vi "Main.vi"() -> (0 "errout":errorcluster caption="error out")   [LabVIEW 2020]
uses:
  <vilib>/MakerHub/LINX/Private/Type Defs/LINX Ref.ctl
  <vilib>/MakerHub/LINX/Private/Type Defs/Platform.ctl
  <vilib>/MakerHub/LINX/Private/Type Defs/Interface.ctl
  <vilib>/MakerHub/LINX/Private/Device/Type Defs/LINX Device Config.ctl
  <vilib>/MakerHub/LINX/Private/Device/Type Defs/TCP Config.ctl
  <vilib>/MakerHub/LINX/Private/Device/Type Defs/Channels.ctl
  ctrl glo/nav.ctl
  <userlib>/Alex Log/Log_ligne.ctl
  ctrl glo/VG_progressBar.vi
  SubVi/Param_Sys.vi
  SubVi/Param_Stack.vi
  <instrlib>/IT6000C/IT6000C.lvlib
  <vilib>/MakerHub/LINX/LMH-LINX.lvlib
  <vilib>/MakerHub/LINX/Private/Device/Device.lvlib
panel:
  out "Config Path":string
  out "chaîne concaténée":string
  out "30?":bool=TRUE
  out "DCIR+?":bool=TRUE
  out "network out":path
  out "Ok final":bool
  out "3P4S?":bool=TRUE
  out "VISA OUT":T1
  out "UNO TAK out":T2
  out "Auto?":bool
  out "progression":u8(slide) scale=0.0..100.0
  out "fin":bool
  out "errout":errorcluster caption="sortie d'erreur"
  in  "image":string
  out "Image 2D":picture
  out "Chaîne 2":string
  out "Chaîne":string
  # "V2.3.1"
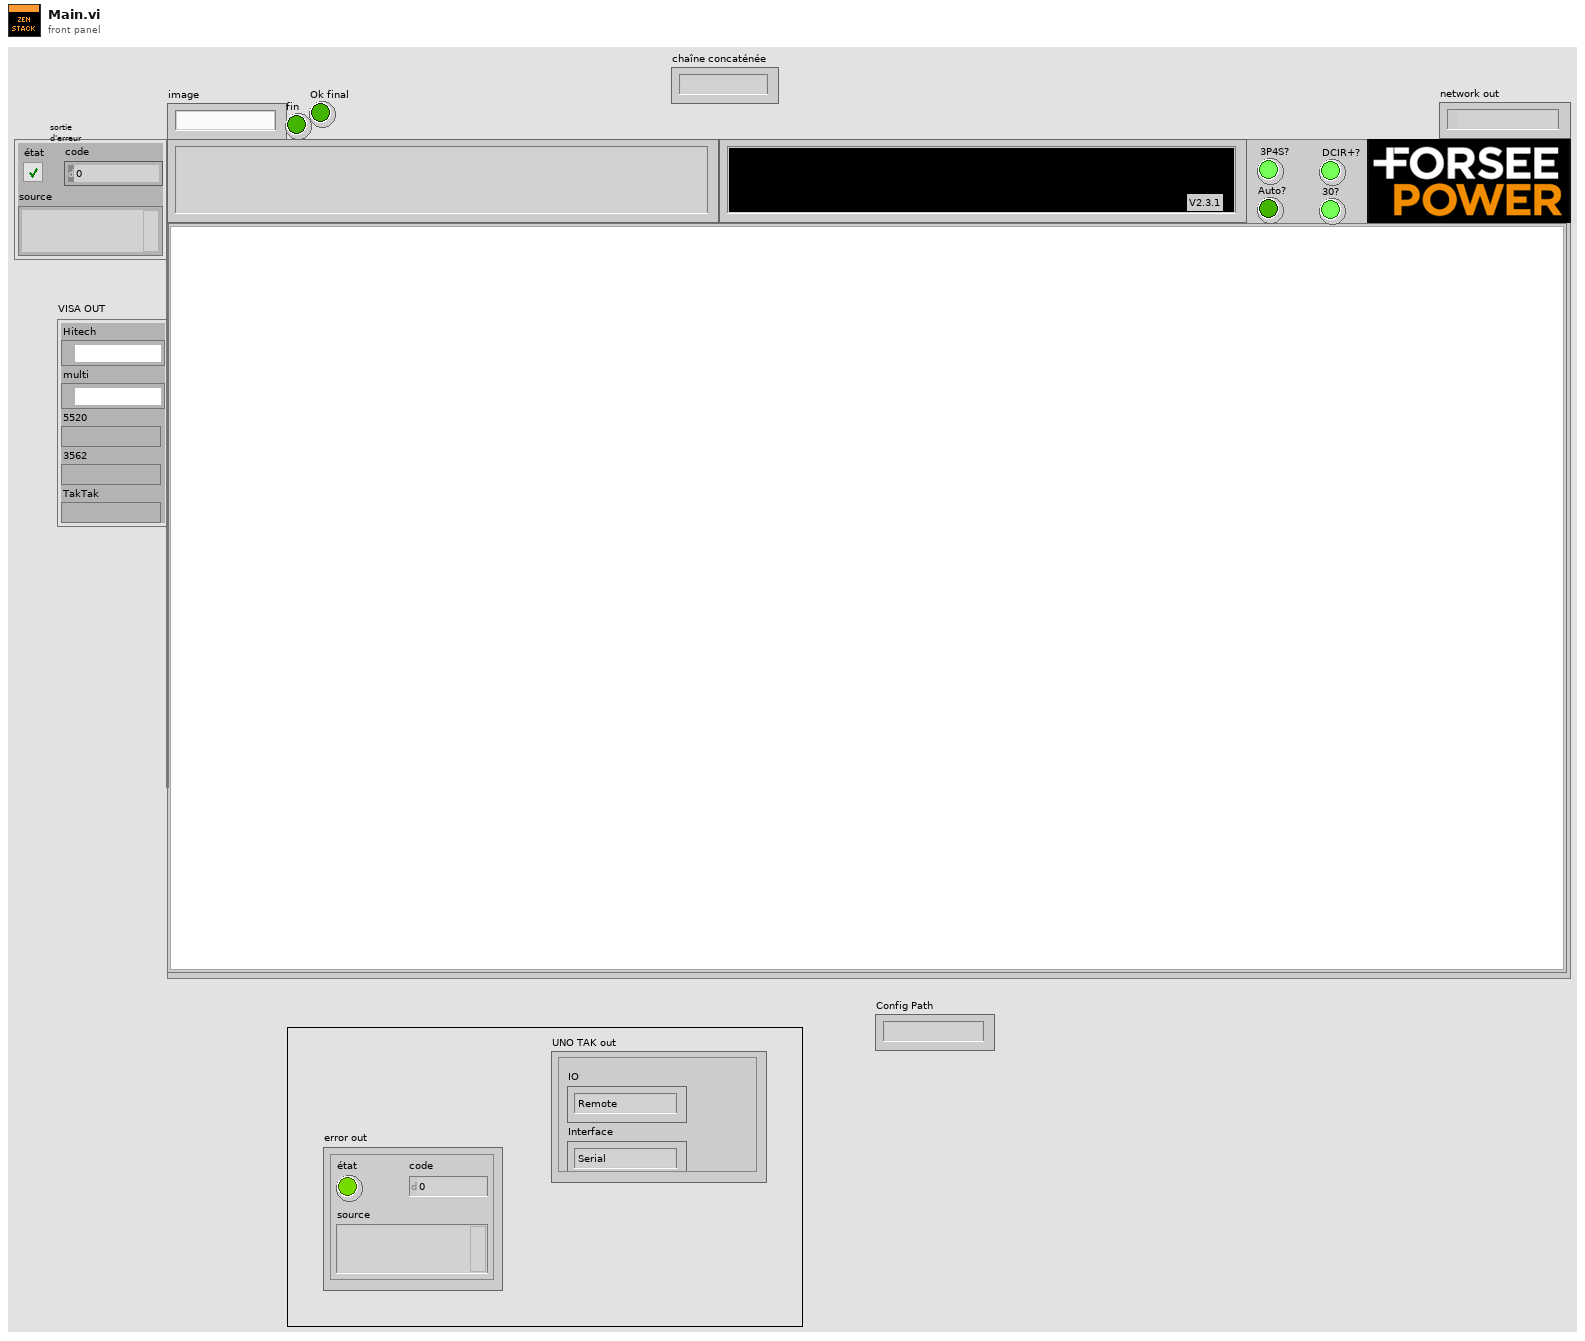
[diagram p1: front panel]
types:
  T1 = cluster{"Hitech":refnum<visa-resource-name>, "multi":refnum<visa-resource-name>, "5520":refnum<visa-resource-name>, "3562":refnum<visa-resource-name>, "TakTak":refnum<visa-resource-name>}
  T2 = typedef "LMH-LINX.lvlib/LINX Ref.ctl" = cluster{"IO":T3, "Interface":T4, "LINX Device Config":T5}
  T3 = typedef "LMH-LINX.lvlib/Platform.ctl" = enum16{"Remote", "Local"}
  T4 = typedef "LMH-LINX.lvlib/Interface.ctl" = enum16{"Serial", "TCP"}
  T5 = typedef "LMH-LINX.lvlib/Device.lvlib/LINX Device Config.ctl" = cluster{"Interface":T4, "COM Port":refnum<visa-resource-name>, "TCP Configuration":T6, "Device Family":u8, "Device ID":u8, "Device Name":string, "TCP Ref":refnum<k5>, "Channels":T7}
  T6 = typedef "LMH-LINX.lvlib/Device.lvlib/TCP Config.ctl" = cluster{"IP Address":string, "Port":u16}
  T7 = typedef "LMH-LINX.lvlib/Channels.ctl" = cluster{"DI":u8[], "DO":u8[], "AI":u8[], "AO":u8[], "PWM":u8[], "QE":u8[], "UART":u8[], "I2C 2":u8[], "SPI":u8[], "CAN":u8[], "Servo":u8[], "AI Ref (V)":dbl, "AI Resolution (Bits)":u8, "AO Ref (V)":dbl, "AO Resolution (Bits)":u8}
  T8 = typedef "nav.ctl" = enum8{"DEM0", "DEM1", "Init", "DEM2", "SCAN", "SECU", "PreDCIR", "OCVACIR", "Montage", "GoInsuPlus", "InsulationBplus", "GoInsuMoins", "InsulationBmoins", "GoDCIR", "DCIR", "Collage PAD", "Demontage", "CLOSE", "extinction", "CRASH"}
  T9 = typedef "Log_ligne.ctl" = enum16{"Def", "Volt V", "Volt mV", "ohm Ohm", "ohm mOhm", "ohm kOhm", "ohm MOhm", "Opérateur", "EPI", "SN"}
  T10 = cluster{"résolution":i16, "resu":dbl, "Type":T9, "Data in":string}
  T11 = cluster{"Baud Rate":u32, "Parity":u16, "Data Bits":u16, "Stop Bits":u16, "Flow Control":u16}
  T12 = cluster{"résolution":i16, "resu":dbl, "Type":T9, "Data in":string}[]
  T13 = cluster{"Cell1 V":sgl, "Cell2 V":sgl, "Cell3 V":sgl, "Cell4 V":sgl, "Cell1 °C":sgl, "Cell2 °C":sgl, "Cell5 V":sgl, "Cell6 V":sgl}
  T14 = typedef "imagedata.ctl" = cluster{"image type":i32, "image depth":i32, "image":u8[], "mask":u8[], "colors":u32[], "Rectangle":cluster{"left":i16, "top":i16, "right":i16, "bottom":i16}}
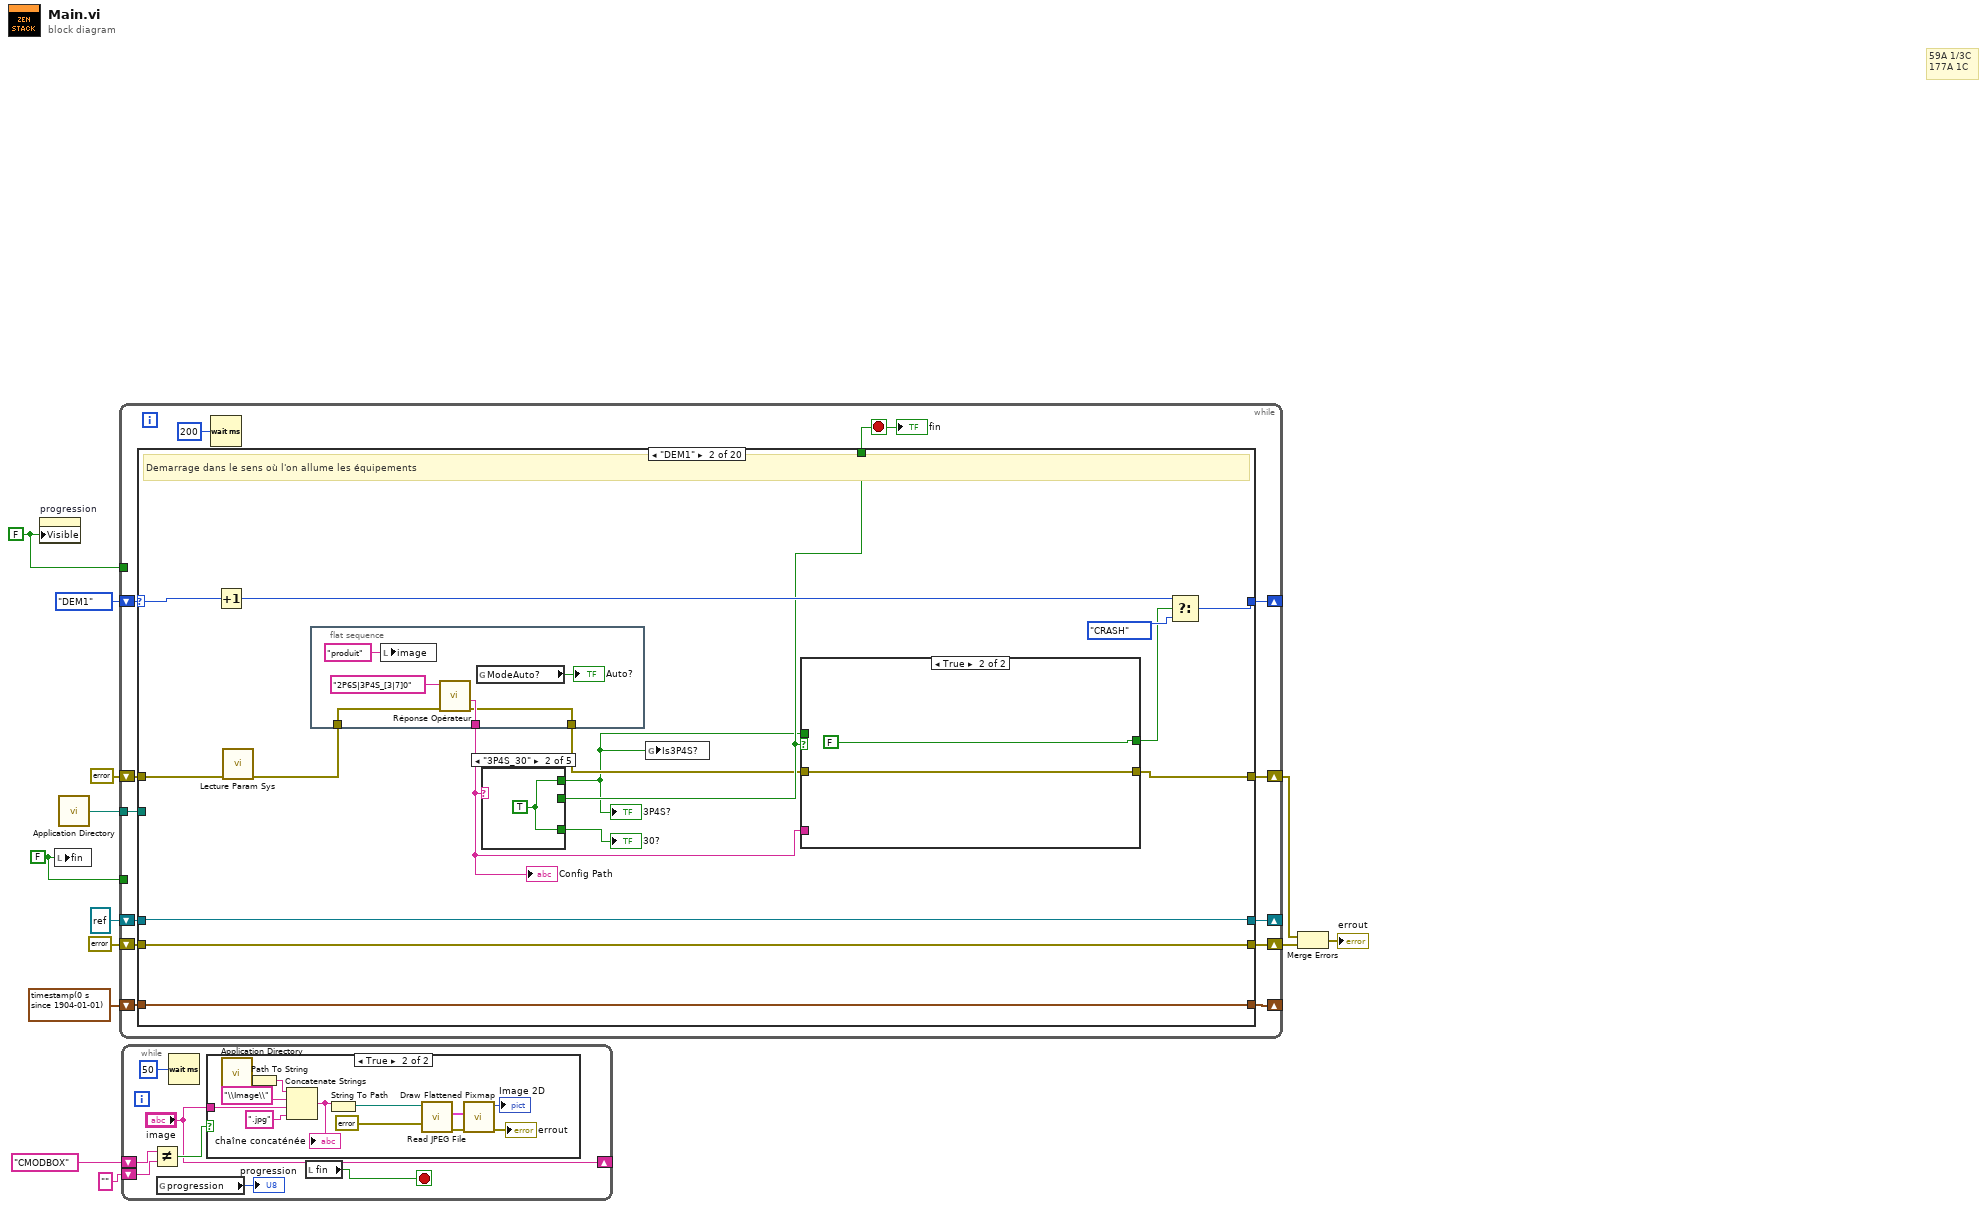
[diagram p0: block diagram]
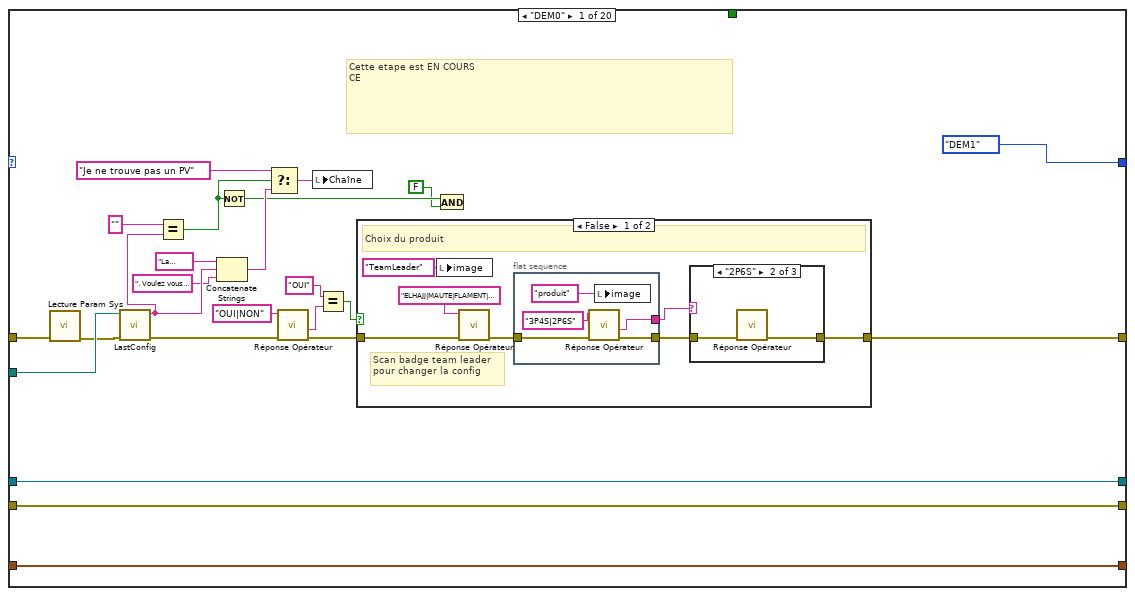
[diagram p3: hidden frame]
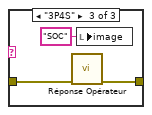
[diagram p5: hidden frame]
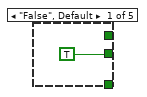
[diagram p7: hidden frame]
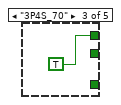
[diagram p8: hidden frame]
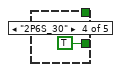
[diagram p9: hidden frame]
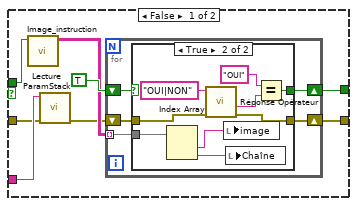
[diagram p11: hidden frame]
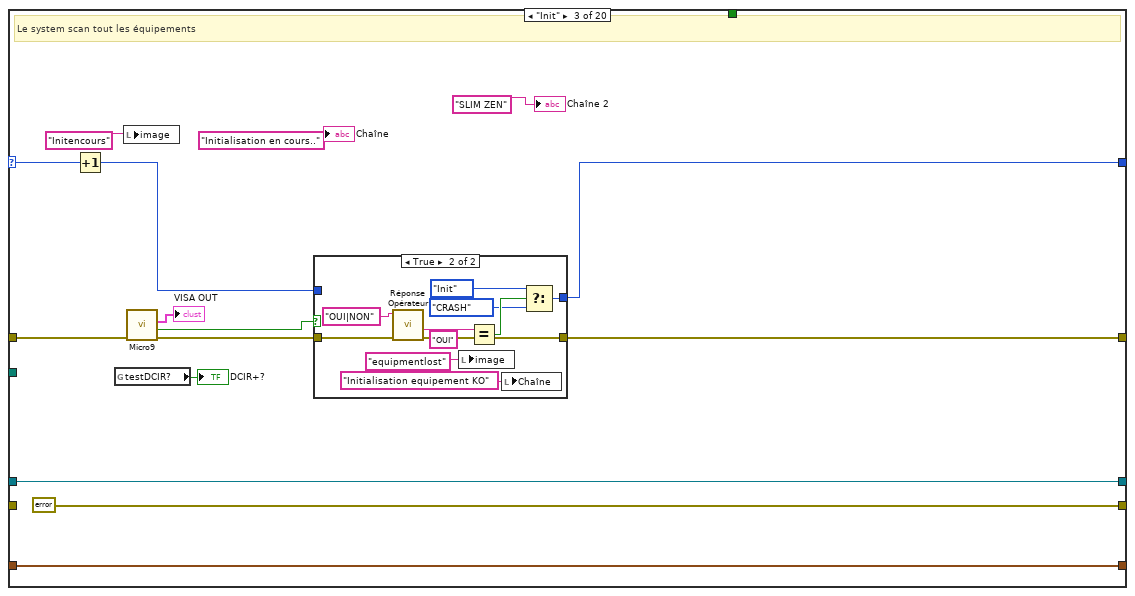
[diagram p13: hidden frame]
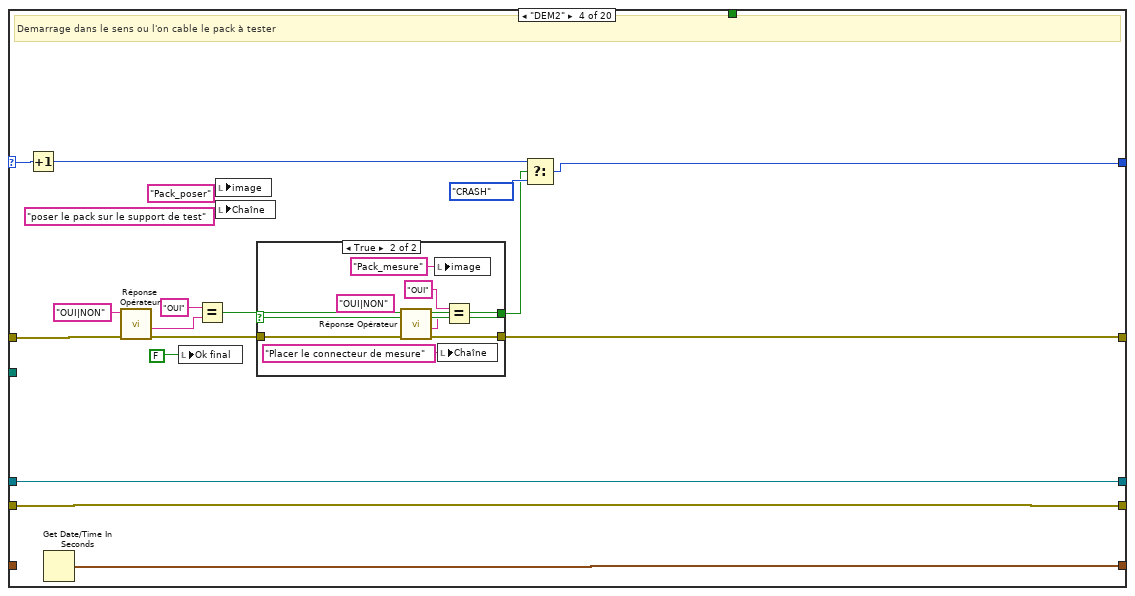
[diagram p15: hidden frame]
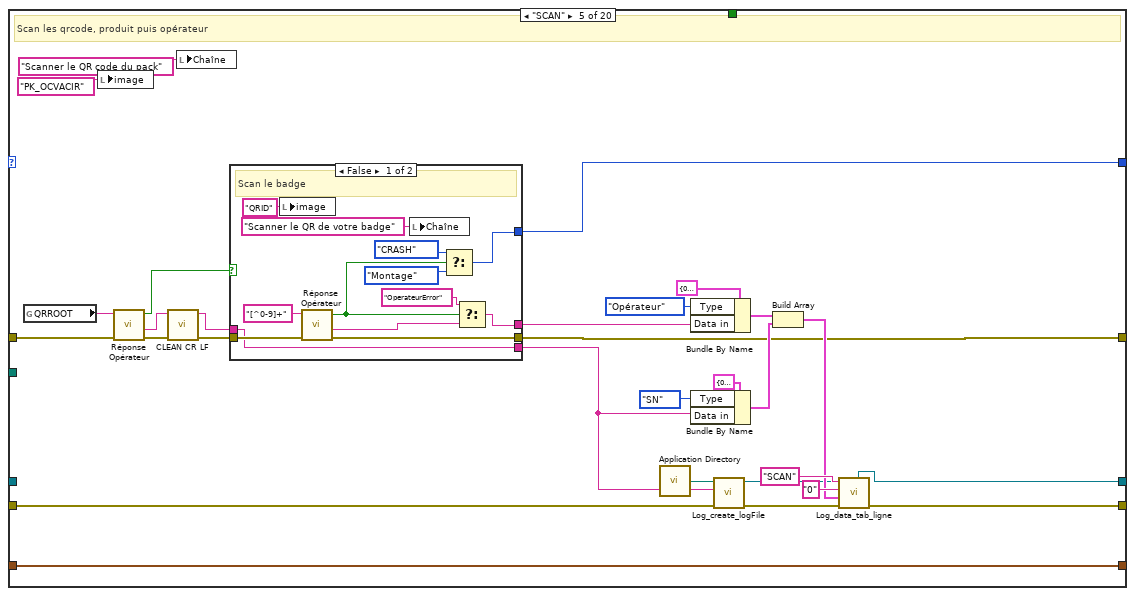
[diagram p17: hidden frame]
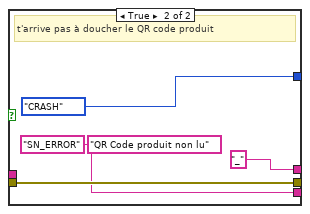
[diagram p18: hidden frame]
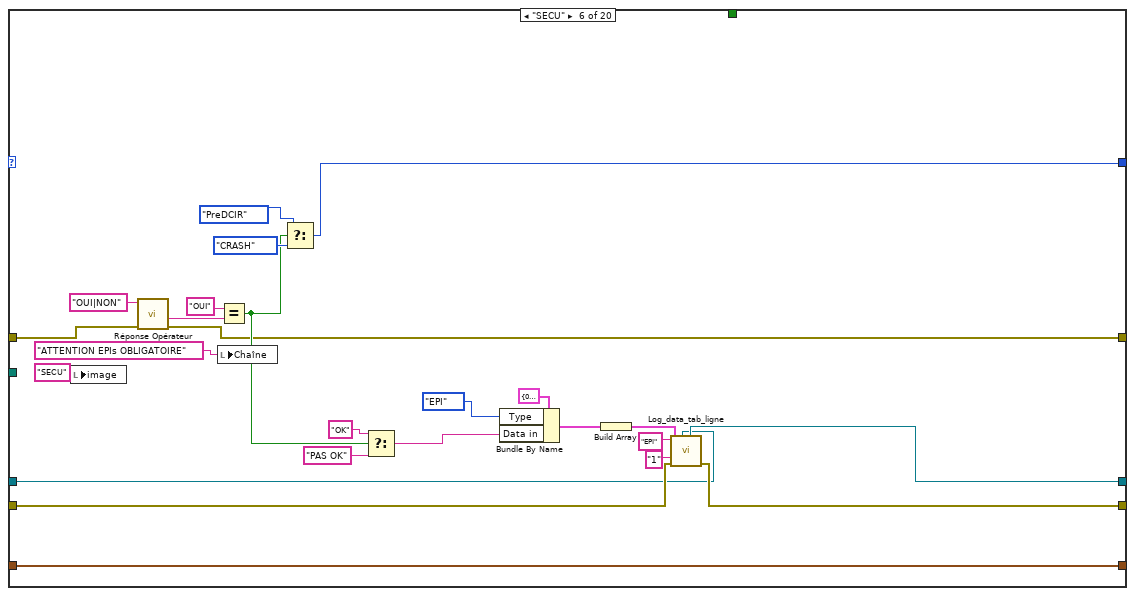
[diagram p19: hidden frame]
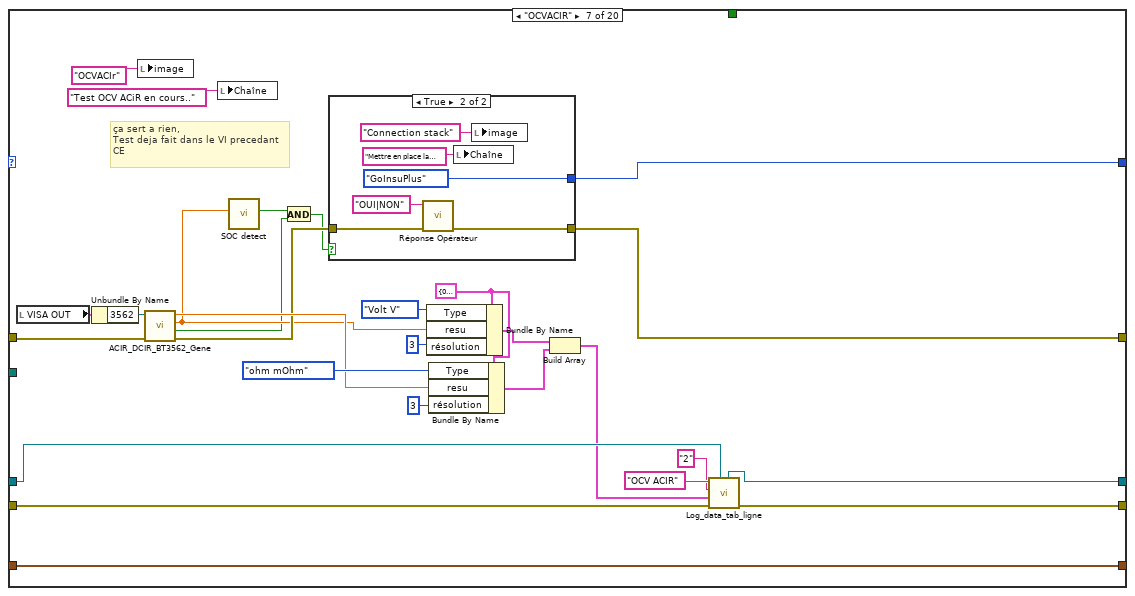
[diagram p20: hidden frame]
diagram:
  w4 = FALSE ("Visible")
  w5 = FALSE ("fin")
  # "59A 1/3C\n177A 1C"
  n1 = property on="progression" class="Slide (strict)"("Visible"=w4) -> ()  [unwired: 2 in, 2 out]
  n2 = local write "fin"(w5) -> ()
  n3 = call <vilib>:"Application Directory.vi"() -> ("Application Directory"=w1:path)
  n4 = while {
    shift-right: [w15] -> w13
    shift-left: errorcluster {"status"=FALSE, "code"=0, "source"=""} ("errout") -> [w25]
    shift-right: [w21] -> _
    shift-left: refnum<file> refnum ("refnum en sortie") -> [w24]
    shift-right: [w22] -> w11
    shift-left: errorcluster {"status"=FALSE, "code"=0, "source"=""} ("errout") -> [w23]
    shift-right: [w19] -> _
    shift-left: timestamp(0 s since 1904-01-01) ("seconds since 1Jan1904") -> [w18]
    shift-right: [w16] -> _
    shift-left: nav."DEM1" -> [w17]
    tunnel: w5 -> [_]
    tunnel: w4 -> [_]
    tunnel: w1 -> [w14]
    stop <- w20 stop-if-true
    n5 = case shown="\"DEM1\"" w17 {
      selector: w17 -> [_ w85 w134 w166 _ _ _ _ _ _ w369 w418 w439 _ w574 _ _ _ _ _]
      tunnel: [_ w76 _ _ _ _ _ _ _ _ _ _ _ _ _ _ TRUE w668 _ _] -> w20
      tunnel: w25 -> [w35 w70 w128 w164 w178 w241 w274 w293 w310 w337 w363 w400 w438 w459 w566 w626 w638 w649 w676 w721]
      tunnel: w24 -> [w48 w84 w133 w154 _ w231 w270 w296 w307 w341 w367 w406 w441 w488 w569 w636 w643 w664 w675 w713]
      tunnel: w23 -> [w49 w83 _ w155 w205 w239 w272 w297 w309 w343 w368 w407 w443 w491 w573 w637 w642 w665 w674 w716]
      tunnel: [w49 w83 errorcluster {"status"=FALSE, "code"=0, "source"=""} ("error out") w155 w190 w238 w271 w297 w308 w342 w366 w408 w442 w490 w573 w609 w642 w648 w674 w715] -> w22
      tunnel: [w48 w84 w133 w154 w189 w240 w269 w296 w306 w340 w365 w405 w440 w487 w569 refnum<file> refnum ("refnum en sortie") w643 refnum<file> refnum ("refnum en sortie") w675 w714] -> w21
      tunnel: [w50 w82 w125 w152 w204 w247 w268 w295 w301 w354 w364 w419 w444 w484 w572 w615 w641 w651 w673 w717] -> w19
      tunnel: w18 -> [w50 w82 w125 _ w204 w247 w268 w295 w301 w354 w364 w419 w444 w484 w572 w615 w641 w651 w673 w717]
      tunnel: [nav."DEM1" w79 w131 w165 w181 w226 w273 nav."PreDCIR" w300 w351 w362 w415 w437 nav."Demontage" w575 w628 nav."CRASH" nav."CRASH" w677 w718] -> w16
      tunnel: [w39 w77 w123 w150 w182 w224 w267 w293 w299 w332 w361 w395 w426 w462 w558 w611 w638 w649 w670 w710] -> w15
      tunnel: w14 -> [w47 _ _ _ _ _ _ _ _ w329 _ w393 _ _ _ _ _ _ _ _]
      frame "DEM0" {
        # "Cette etape est EN COURS\nCE"
        n6 = call "Lecture Param Sys.vi"("errin"=w35) -> ("error out"=w36:errorcluster)  [unwired: 10 in]
        n7 = call "LastConfig.vi"("errin"=w36, "Application Directory"=w47) -> ("error out"=w32:errorcluster, "Derniere Config"=w42:string)  [unwired: 8 in]
        n8 = Equal?(x="", y=w42) -> (x = y?=w38:bool)
        n9 = Concatenate Strings("La derniere config est : " ("f"), w42, ". Voulez vous rester sur cette config ?" ("f")) -> (w44:string)
        n10 = Not(x=w38) -> (.not. x?=w37:bool)
        n11 = Select(t="Je ne trouve pas un PV" ("x"), s=w38, f=w44) -> (s? t:f=w41:string)
        n12 = call "Réponse Opérateur.vi"("errin"=w32, "expression régulière"="OUI|NON" ("image")) -> ("errout"=w30:errorcluster, "toute l'expression"=w28:string)  [unwired: 7 in, 1 out]
        n13 = local write "Chaîne"(w41) -> ()
        n14 = Equal?(x="OUI", y=w28) -> (x = y?=w27:bool)
        n15 = case shown="False" w27 {
          tunnel: w30 -> [w57 w69]
          tunnel: [w52 w69] -> w39
          frame False {
            # "Scan badge team leader pour changer la config"
            # "Choix du produit"
            n16 = local write "image"("TeamLeader" ("image")) -> ()
            n17 = call "Réponse Opérateur.vi"("errin"=w57, "expression régulière"="ELHAJJ|MAUTE|FLAMENT|MOURA CAEIRO|LECLERE") -> ("errout"=w54:errorcluster)  [unwired: 7 in, 2 out]
            n18 = flat-sequence {
              tunnel: w54 -> [w67]
              tunnel: [w66] -> w53
              tunnel: [w64] -> w51
              frame #0 {
                n19 = call "Réponse Opérateur.vi"("errin"=w67, "expression régulière"="3P4S|2P6S" ("image")) -> ("errout"=w66:errorcluster, "toute l'expression"=w64:string)  [unwired: 7 in, 1 out]
                n20 = local write "image"("produit" ("image")) -> ()
              }
            }
            n21 = case shown="\"2P6S\"" w51 {
              tunnel: w53 -> [w58 w60 w63]
              tunnel: [w58 w59 w62] -> w52
              frame "NULL", Default {
              }
              frame "2P6S" {
                n22 = call "Réponse Opérateur.vi"("errin"=w60) -> ("errout"=w59:errorcluster)  [unwired: 8 in, 2 out]
              }
              frame "3P4S" {
                n23 = call "Réponse Opérateur.vi"("errin"=w63) -> ("errout"=w62:errorcluster)  [unwired: 8 in, 2 out]
                n24 = local write "image"("SOC" ("image")) -> ()
              }
            }
          }
          frame True {
            # "On change pas la config"
          }
        }
        n25 = And(x=w37, y=FALSE) -> ()  [unwired: 1 out]
      }
      frame "DEM1" {
        # "Demarrage dans le sens où l'on allume les équipements"
        n26 = Increment(x=w85) -> (x+1=w80:T8)
        n27 = call "Lecture Param Sys.vi"("errin"=w70) -> ("error out"=w71:errorcluster)  [unwired: 10 in]
        n28 = flat-sequence {
          tunnel: w71 -> [w93]
          tunnel: [w92] -> w73
          tunnel: [w90] -> w74
          frame #0 {
            n29 = local write "image"("produit" ("image")) -> ()
            n30 = call "Réponse Opérateur.vi"("errin"=w93, "expression régulière"="2P6S|3P4S_[3|7]0") -> ("errout"=w90:errorcluster, "toute l'expression"=w92:string)  [unwired: 7 in, 1 out]
            n31 = global read "Param_Sys.vi" "ModeAuto?"() -> (→"Auto?":bool)
          }
        }
        n32 = case shown="\"3P4S_30\"" w73 {
          tunnel: [_ w87 TRUE _ _] -> w72
          tunnel: [TRUE _ _ _ _] -> w76
          tunnel: [_ w87 _ TRUE _] -> w75
          frame "False", Default {
          }
          frame "3P4S_30" {
            w87 = TRUE
          }
          frame "3P4S_70" {
          }
          frame "2P6S_30" {
          }
          frame "2P6S_70" {
          }
        }
        "3P4S?" <- w72
        "30?" <- w75
        n33 = global write "Param_Stack.vi" "Is3P4S?"(w72) -> ()
        n34 = case shown="True" w76 {
          tunnel: [w102 FALSE] -> w78
          tunnel: [w101 w120] -> w77
          tunnel: w74 -> [w98 w120]
          tunnel: w73 -> [w99 _]
          tunnel: w72 -> [w96 _]
          frame False {
            n35 = call "Image_instruction.vi"("3P4S?"=w96) -> ("Array"=w100:string[][])  [unwired: 10 in]
            n36 = call "Lecture ParamStack.vi"("errin"=w98, "varriante"=w99) -> ("error out"=w97:errorcluster)  [unwired: 9 in]
            n37 = for {
              tunnel: w100 -> [w108] mode=indexing
              shift-right: [w107] -> w102
              shift-left: TRUE -> [w106]
              shift-right: [w105] -> w101
              shift-left: w97 -> [w104]
              n38 = case shown="True" w106 {
                selector: w106 -> [w110 _]
                tunnel: w108 -> [_ w116]
                tunnel: [w110 w113] -> w107
                tunnel: [w109 w112] -> w105
                tunnel: w104 -> [w109 w111]
                frame False {
                }
                frame True {
                  n39 = Index Array(array=w116) -> (element #1=w115:string, element #2=w114:string)  [unwired: 2 in]
                  n40 = call "Réponse Opérateur.vi"("errin"=w111, "expression régulière"="OUI|NON") -> ("errout"=w112:errorcluster, "toute l'expression"=w117:string)  [unwired: 7 in, 1 out]
                  n41 = local write "image"(w115) -> ()
                  n42 = local write "Chaîne"(w114) -> ()
                  n43 = Equal?(x="OUI", y=w117) -> (x = y?=w113:bool)
                }
              }
            }
          }
          frame True {
          }
        }
        n44 = Select(t=w80, s=w78, f=nav."CRASH") -> (s? t:f=w79:T8)
        "Config Path" <- w73
      }
      frame "Init" {
        # "Le system scan tout les équipements"
        n45 = Increment(x=w134) -> (x+1=w130:T8)
        n46 = global read "Param_Stack.vi" "testDCIR?"() -> (→"DCIR+?":bool)
        n47 = local write "image"("Initencours") -> ()
        n48 = call "Micro9.vi"("errin"=w128) -> ("errout"=w124:errorcluster, "KO?"=w132:bool, "VISA OUT"=→"VISA OUT":T1)  [unwired: 8 in]
        n49 = case shown="True" w132 {
          tunnel: w124 -> [w138 w139]
          tunnel: [w138 w148] -> w123
          tunnel: w130 -> [w137 _]
          tunnel: [w137 w142] -> w131
          frame False {
          }
          frame True {
            n50 = call "Réponse Opérateur.vi"("errin"=w139, "expression régulière"="OUI|NON") -> ("errout"=w148:errorcluster, "toute l'expression"=w147:string)  [unwired: 7 in, 1 out]
            n51 = local write "image"("equipmentlost") -> ()
            n52 = Equal?(x=w147, y="OUI") -> (x = y?=w145:bool)
            n53 = local write "Chaîne"("Initialisation equipement KO" ("Chaîne")) -> ()
            n54 = Select(t=nav."Init", s=w145, f=nav."CRASH") -> (s? t:f=w142:T8)
          }
        }
        "Chaîne" <- "Initialisation en cours.." ("Chaîne")
        "Chaîne 2" <- "SLIM ZEN" ("Chaîne 2")
      }
      frame "DEM2" {
        # "Demarrage dans le sens ou l'on cable le pack à tester"
        n55 = Increment(x=w166) -> (x+1=w167:T8)
        n56 = Get Date/Time In Seconds() -> (seconds since 1Jan1904=w152:timestamp)
        n57 = call "Réponse Opérateur.vi"("errin"=w164, "expression régulière"="OUI|NON") -> ("errout"=w157:errorcluster, "toute l'expression"=w162:string)  [unwired: 7 in, 1 out]
        n58 = local write "Ok final"(FALSE ("OK?")) -> ()
        n59 = Equal?(x="OUI", y=w162) -> (x = y?=w156:bool)
        n60 = local write "image"("Pack_poser") -> ()
        n61 = local write "Chaîne"("poser le pack sur le support de test" ("chaîne")) -> ()
        n62 = case shown="True" w156 {
          selector: w156 -> [w169 _]
          tunnel: w157 -> [w168 w170]
          tunnel: [w169 w173] -> w151
          tunnel: [w168 w176] -> w150
          frame False {
          }
          frame True {
            n63 = call "Réponse Opérateur.vi"("errin"=w170, "expression régulière"="OUI|NON") -> ("errout"=w176:errorcluster, "toute l'expression"=w174:string)  [unwired: 7 in, 1 out]
            n64 = local write "image"("Pack_mesure") -> ()
            n65 = local write "Chaîne"("Placer le connecteur de mesure" ("chaîne")) -> ()
            n66 = Equal?(x="OUI", y=w174) -> (x = y?=w173:bool)
          }
        }
        n67 = Select(t=w167, s=w151, f=nav."CRASH") -> (s? t:f=w165:T8)
      }
      frame "SCAN" {
        # "Scan les qrcode, produit puis opérateur"
        n68 = global read "Param_Stack.vi" "QRROOT"() -> (w179:string)
        n69 = local write "image"("PK_OCVACIR") -> ()
        n70 = call "Réponse Opérateur.vi"("errin"=w178, "expression régulière"=w179) -> ("errout"=w184:errorcluster, "toute l'expression"=w188:string, "ArrsurErr"=w203:bool)  [unwired: 7 in]
        n71 = call "CLEAN CR LF.vi"("errin"=w184, "in"=w188) -> ("errout"=w183:errorcluster, "out"=w187:string)  [unwired: 8 in]
        n72 = local write "Chaîne"("Scanner le QR code du pack" ("Chaîne")) -> ()
        n73 = case shown="False" w203 {
          tunnel: w183 -> [w209 w222]
          tunnel: [w215 w222] -> w182
          tunnel: [w216 nav."CRASH"] -> w181
          tunnel: w187 -> [w207 _]
          tunnel: [w208 "_" ("toute l'expression")] -> w185
          tunnel: [w207 "SN_ERROR" ("toute l'expression")] -> w186
          frame False {
            # "Scan le badge"
            n74 = local write "image"("QRID") -> ()
            n75 = call "Réponse Opérateur.vi"("errin"=w209, "expression régulière"="[^0-9]+") -> ("errout"=w215:errorcluster, "toute l'expression"=w212:string, "ArrsurErr"=w214:bool)  [unwired: 7 in]
            n76 = local write "Chaîne"("Scanner le QR de votre badge" ("Chaîne")) -> ()
            n77 = Select(t=nav."CRASH", s=w214, f=nav."Montage") -> (s? t:f=w216:T8)
            n78 = Select(t="OperateurError" ("chaîne"), s=w214, f=w212) -> (s? t:f=w208:string)
          }
          frame True {
            (unwired) "QR Code produit non lu" ("toute l'expression")
            # "t'arrive pas à doucher le QR code produit"
          }
        }
        n79 = call <vilib>:"Application Directory.vi"() -> ("Application Directory"=w206:path)
        n80 = Bundle By Name(cluster=T10 {"résolution"=0, "resu"=0.0, "Type"=enum."EPI", "Data in"="MOI"} ("data"), "Type"=Log_ligne."Opérateur", "Data in"=w185) -> (w195:T10)
        n81 = Bundle By Name(cluster=T10 {"résolution"=0, "resu"=0.0, "Type"=enum."EPI", "Data in"="MOI"} ("data"), "Type"=Log_ligne."SN", "Data in"=w186) -> (w194:T10)
        n82 = call <userlib>:"Log_create_logFile.vi"("errin"=w205, "toute l'expression"=w186, "Application Directory"=w206) -> ("sortie d'erreur"=w191:errorcluster, "Fichier à flux d'octets en sortie"=w192:refnum<file>)  [unwired: 7 in]
        n83 = Build Array(w195, w194) -> (w193:T12)
        n84 = call <userlib>:"Log_data_tab_ligne.vi"("in"=w192, "errin"=w191, "Tableau"=w193, "test number"="0", "test name"="SCAN") -> ("sortie d'erreur"=w190:errorcluster, "refnum en sortie"=w189:refnum<file>)  [unwired: 5 in]
      }
      frame "SECU" {
        n85 = local write "image"("SECU") -> ()
        n86 = call "Réponse Opérateur.vi"("errin"=w241, "expression régulière"="OUI|NON") -> ("errout"=w224:errorcluster, "toute l'expression"=w244:string)  [unwired: 7 in, 1 out]
        n87 = local write "Chaîne"("ATTENTION EPIs OBLIGATOIRE" ("Chaîne")) -> ()
        n88 = Equal?(x="OUI", y=w244) -> (x = y?=w230:bool)
        n89 = Select(t=nav."PreDCIR", s=w230, f=nav."CRASH") -> (s? t:f=w226:T8)
        n90 = Select(t="OK", s=w230, f="PAS OK" ("cas faux")) -> (s? t:f=w227:string)
        n91 = Bundle By Name(cluster=T10 {"résolution"=0, "resu"=0.0, "Type"=enum."EPI", "Data in"="MOI"} ("data"), "Type"=Log_ligne."EPI", "Data in"=w227) -> (w233:T10)
        n92 = Build Array(w233) -> (w232:T12)
        n93 = call <userlib>:"Log_data_tab_ligne.vi"("in"=w231, "errin"=w239, "Tableau"=w232, "test number"="1", "test name"="EPI") -> ("sortie d'erreur"=w238:errorcluster, "refnum en sortie"=w240:refnum<file>)  [unwired: 5 in]
      }
      frame "OCVACIR" {
        w257 = T10 {"résolution"=0, "resu"=0.0, "Type"=enum."EPI", "Data in"="MOI"} ("data")
        # "ça sert a rien,\nTest deja fait dans le VI precedant\nCE"
        n94 = local read "VISA OUT"() -> (w255:T1)
        n95 = Unbundle By Name(w255) -> ("3562"=w254:refnum<visa-resource-name>)
        n96 = local write "image"("OCVACIr") -> ()
        n97 = call <userlib>:"ACIR_DCIR_BT3562_Gene.vi"("errin"=w274, "VISAin"=w254) -> ("errout"=w253:errorcluster, "OK?"=w250:bool, "V"=w252:dbl, "R"=w256:dbl)  [unwired: 3 in, 3 out]
        n98 = local write "Chaîne"("Test OCV ACiR en cours.." ("Chaîne")) -> ()
        n99 = call "SOC detect.vi"("Vmeasure"=w252) -> ("testresult"=w251:bool)  [unwired: 9 in, 1 out]
        n100 = And(x=w251, y=w250) -> (x .and. y?=w249:bool)
        n101 = case shown="True" w249 {
          tunnel: w253 -> [w277 w291]
          tunnel: [w282 w290] -> w267
          tunnel: [w279 nav."GoInsuPlus"] -> w273
          frame False {
            n102 = local write "image"("Refaire") -> ()
            n103 = call "Réponse Opérateur.vi"("errin"=w277, "expression régulière"="OUI|NON") -> ("errout"=w282:errorcluster, "toute l'expression"=w284:string)  [unwired: 7 in, 1 out]
            n104 = Equal?(x=w284, y="OUI") -> (x = y?=w285:bool)
            n105 = Select(t=nav."OCVACIR", s=w285, f=nav."CRASH") -> (s? t:f=w279:T8)
          }
          frame True {
            n106 = call "Réponse Opérateur.vi"("errin"=w291, "expression régulière"="OUI|NON") -> ("errout"=w290:errorcluster)  [unwired: 7 in, 2 out]
            n107 = local write "Chaîne"("Mettre en place la cloche" ("chaîne")) -> ()
            n108 = local write "image"("Connection stack") -> ()
          }
        }
        n109 = Bundle By Name(cluster=w257, "Type"=Log_ligne."Volt V", "resu"=w252, "résolution"=i16 3) -> (w265:T10)
        n110 = Bundle By Name(cluster=w257, "Type"=Log_ligne."ohm mOhm", "resu"=w256, "résolution"=i16 3) -> (w258:T10)
        n111 = Build Array(w265, w258) -> (w261:T12)
        n112 = call <userlib>:"Log_data_tab_ligne.vi"("in"=w270, "errin"=w272, "Tableau"=w261, "test number"="2", "test name"="OCV ACIR") -> ("sortie d'erreur"=w271:errorcluster, "refnum en sortie"=w269:refnum<file>)  [unwired: 5 in]
      }
      frame "Montage" {
      }
      frame "GoInsuPlus" {
        n113 = local read "Auto?"() -> (w311:bool)
        n114 = Select(t="InsuPlusAUTO", s=w311, f="InsuPlus") -> (s? t:f=w304:string)
        n115 = Select(t="Le PC commute sur l'isolement + ...", s=w311, f="Se mettre sur Isolement +") -> (s? t:f=w303:string)
        n116 = local write "image"(w304) -> ()
        n117 = local write "Chaîne"(w303) -> ()
        n118 = case shown="True" w311 {
          tunnel: w310 -> [w318 w328]
          tunnel: [w317 w326] -> w299
          tunnel: nav."InsulationBplus" -> [w316 w324]
          tunnel: [w316 w322] -> w300
          frame False {
            n119 = call "Réponse Opérateur.vi"("errin"=w318, "expression régulière"="OUI") -> ("errout"=w317:errorcluster)  [unwired: 7 in, 2 out]
          }
          frame True {
            # "Le PC switch le TakTak en isolement +"
            n120 = local read "VISA OUT"() -> (w321:T1)
            n121 = Unbundle By Name(w321) -> ("TakTak"=w320:refnum<visa-resource-name>)
            n122 = call "SET ISO BAT PLUS.vi"("Error In"=w328, "port tak"=w320) -> ("Error Out"=w326:errorcluster, "UNO TAK out"=→"UNO TAK out":T2)  [unwired: 8 in]
            n123 = Unbundle By Name(w326) -> ("status"=w325:bool)
            n124 = Select ("Sélectionner")(t=nav."CRASH" ("cas vrai"), s=w325, f=w324) -> (s? t:f=w322:T8)
          }
        }
        n125 = Concatenate Strings(w304, "\r\n") -> (w305:string)
        n126 = Write to Text File ("Écrire dans un fichier texte")(file (use dialog)=w307, text=w305, error in=w309) -> (refnum out=w306:refnum<file>, error out=w308:errorcluster)  [unwired: 1 in, 1 out]
      }
      frame "InsulationBplus" {
        n127 = flat-sequence {
          tunnel: w337 -> [w359]
          tunnel: [w359] -> w349
          frame #0 {
            n128 = local write "image"("TestEnCoursSecu") -> ()
          }
        }
        n129 = local read "VISA OUT"() -> (w334:T1)
        n130 = local write "Chaîne"("Test insulation Bat + en cours.." ("Chaîne")) -> ()
        n131 = Unbundle By Name(w334) -> ("5520"=w333:refnum<visa-resource-name>)
        n132 = call <userlib>:"Insulation_ST5520.vi"("errin"=w349, "chemin de base"=w329, "Refnum VISA en entrée"=w333) -> ("error out"=w336:errorcluster, "PASS?"=w352:bool, "R iso(MOhm)"=w331:dbl)  [unwired: 6 in]
        n133 = Bundle By Name(cluster=T10 {"résolution"=0, "resu"=0.0, "Type"=enum."EPI", "Data in"="MOI"} ("data"), "Type"=Log_ligne."ohm MOhm", "resu"=w331, "résolution"=i16 0) -> (w346:T10)
        n134 = Build Array(w346) -> (w338:T12)
        n135 = local read "Auto?"() -> (w335:bool)
        n136 = case shown="True" w335 {
          tunnel: w336 -> [w355 w358]
          tunnel: [w355 w357] -> w332
          frame False {
          }
          frame True {
            n137 = local read "UNO TAK out"() -> (w356:T2)
            n138 = call "Close TakTak.vi"("errin"=w358, "UNO Tak in"=w356) -> ("Error Out"=w357:errorcluster)  [unwired: 9 in]
          }
        }
        n139 = call <userlib>:"Log_data_tab_ligne.vi"("in"=w341, "errin"=w343, "Tableau"=w338, "test number"="3", "test name"="BAT+" ("chaîne")) -> ("sortie d'erreur"=w342:errorcluster, "refnum en sortie"=w340:refnum<file>)  [unwired: 5 in]
        n140 = Select(t=nav."GoInsuMoins", s=w352, f=nav."Demontage") -> (s? t:f=w351:T8)
      }
      frame "GoInsuMoins" {
        n141 = Increment(x=w369) -> (x+1=w370:T8)
        n142 = local read "Auto?"() -> (w375:bool)
        n143 = Select(t="InsuMoinsAUTO", s=w375, f="InsuMoins") -> (s? t:f=w373:string)
        n144 = Select(t="Le PC commute sur l'isolement - ...", s=w375, f="Se mettre sur Isolement -") -> (s? t:f=w372:string)
        n145 = local write "image"(w373) -> ()
        n146 = local write "Chaîne"(w372) -> ()
        n147 = Concatenate Strings(w373, "\r\n") -> (w374:string)
        n148 = Write to Text File ("Écrire dans un fichier texte")(file (use dialog)=w367, text=w374, error in=w368) -> (refnum out=w365:refnum<file>, error out=w366:errorcluster)  [unwired: 1 in, 1 out]
        n149 = case shown="True" w375 {
          tunnel: w363 -> [w382 w392]
          tunnel: [w381 w391] -> w361
          tunnel: w370 -> [w380 w389]
          tunnel: [w380 w387] -> w362
          frame False {
            n150 = call "Réponse Opérateur.vi"("errin"=w382, "expression régulière"="OUI") -> ("errout"=w381:errorcluster)  [unwired: 7 in, 2 out]
          }
          frame True {
            # "Le PC switch le TakTak en isolement -"
            n151 = local read "VISA OUT"() -> (w384:T1)
            n152 = Unbundle By Name(w384) -> ("TakTak"=w385:refnum<visa-resource-name>)
            n153 = call "SET ISO BAT MOINS.vi"("Error In"=w392, "Port tak"=w385) -> ("Error Out"=w391:errorcluster, "UNO TAK out"=w386:T2)  [unwired: 8 in]
            n154 = local write "UNO TAK out"(w386) -> ()
            n155 = Unbundle By Name(w391) -> ("status"=w390:bool)
            n156 = Select ("Sélectionner")(t=nav."CRASH" ("cas vrai"), s=w390, f=w389) -> (s? t:f=w387:T8)
          }
        }
      }
      frame "InsulationBmoins" {
        n157 = flat-sequence {
          tunnel: [w424] -> w412
          tunnel: w400 -> [w424]
          frame #0 {
            n158 = local write "image"("TestEnCoursSecu") -> ()
          }
        }
        n159 = Increment(x=w418) -> (x+1=w416:T8)
        n160 = local read "VISA OUT"() -> (w397:T1)
        n161 = local write "Chaîne"("Test insulation Bat - en cours.." ("Chaîne")) -> ()
        n162 = Unbundle By Name(w397) -> ("5520"=w396:refnum<visa-resource-name>)
        n163 = call <userlib>:"Insulation_ST5520.vi"("errin"=w412, "chemin de base"=w393, "Refnum VISA en entrée"=w396) -> ("error out"=w399:errorcluster, "PASS?"=w414:bool, "R iso(MOhm)"=w394:dbl)  [unwired: 6 in]
        n164 = Select(t=w416, s=w414, f=nav."Demontage") -> (s? t:f=w415:T8)
        n165 = Bundle By Name(cluster=T10 {"résolution"=0, "resu"=0.0, "Type"=enum."EPI", "Data in"="MOI"} ("data"), "Type"=Log_ligne."ohm MOhm", "resu"=w394, "résolution"=i16 0) -> (w409:T10)
        n166 = local read "Auto?"() -> (w398:bool)
        n167 = Build Array(w409) -> (w404:T12)
        n168 = case shown="False" w398 {
          tunnel: w399 -> [w420 w423]
          tunnel: [w420 w422] -> w395
          frame False {
          }
          frame True {
            n169 = local read "UNO TAK out"() -> (w421:T2)
            n170 = call "Close TakTak.vi"("errin"=w423, "UNO Tak in"=w421) -> ("Error Out"=w422:errorcluster)  [unwired: 9 in]
          }
        }
        n171 = call <userlib>:"Log_data_tab_ligne.vi"("in"=w406, "errin"=w407, "Tableau"=w404, "test number"="4", "test name"="BAT-" ("chaîne")) -> ("sortie d'erreur"=w408:errorcluster, "refnum en sortie"=w405:refnum<file>)  [unwired: 5 in]
      }
      frame "GoDCIR" {
        n172 = Increment(x=w439) -> (x+1=w436:T8)
        n173 = local read "Auto?"() -> (w427:bool)
        n174 = Select(t="Mode DCIRAUTO", s=w427, f="Mode DCIR") -> (s? t:f=w434:string)
        n175 = Select(t="Le PC commute sur DCIR...", s=w427, f="Se mettre sur DCIR") -> (s? t:f=w435:string)
        n176 = local write "image"(w434) -> ()
        n177 = local write "Chaîne"(w435) -> ()
        n178 = case shown="True" w427 {
          tunnel: [w447 w452] -> w426
          tunnel: w436 -> [w446 w456]
          tunnel: [w446 w454] -> w437
          tunnel: w438 -> [w445 w453]
          frame False {
            n179 = call "Réponse Opérateur.vi"("errin"=w445, "expression régulière"="OUI") -> ("errout"=w447:errorcluster)  [unwired: 7 in, 2 out]
          }
          frame True {
            # "Le PC switch le TakTak en DCIR"
            n180 = local read "VISA OUT"() -> (w450:T1)
            n181 = Unbundle By Name(w450) -> ("TakTak"=w449:refnum<visa-resource-name>)
            n182 = call "SET DCIR.vi"("Error In"=w453, "Port Tak"=w449) -> ("Error Out"=w452:errorcluster, "UNO TAK out"=w451:T2)  [unwired: 8 in]
            n183 = local write "UNO TAK out"(w451) -> ()
            n184 = Unbundle By Name(w452) -> ("status"=w457:bool)
            n185 = Select ("Sélectionner")(t=nav."CRASH" ("cas vrai"), s=w457, f=w456) -> (s? t:f=w454:T8)
          }
        }
        n186 = Concatenate Strings(w434, "\r\n") -> (w433:string)
        n187 = Write to Text File ("Écrire dans un fichier texte")(file (use dialog)=w441, text=w433, error in=w443) -> (refnum out=w440:refnum<file>, error out=w442:errorcluster)  [unwired: 1 in, 1 out]
      }
      frame "DCIR" {
        n188 = local read "3P4S?"() -> (w469:bool)
        n189 = local read "VISA OUT"() -> (w478:T1)
        n190 = global read "Param_Stack.vi" "Current"() -> (w461:dbl)
        n191 = global write "VG_progressBar.vi" "progression"(u8 0 ("progression")) -> ()
        n192 = local write "image"("DCIR" ("Chaîne")) -> ()
        n193 = Unbundle By Name(w478) -> ("Hitech"=w477:refnum<visa-resource-name>)
        n194 = property on="progression" class="Slide (strict)"(error in=w459, "Visible"=TRUE) -> (error out=w464:errorcluster)  [unwired: 1 in, 1 out]
        n195 = local write "Chaîne"("Test DCIR: Lecture des Cell" ("Chaîne")) -> ()
        n196 = Negate(x=w461) -> (-x=w460:dbl)
        n197 = call <instrlib>:"Initialize.vi"("Serial Configuration"=T11 {"Baud Rate"=9600, "Parity"=0, "Data Bits"=8, "Stop Bits"=10, "Flow Control"=0} ("Sérialconf"), "error in (no error)"=w459, "VISA resource name"=w477) -> ("error out"=w495:errorcluster, "VISA resource name out"=w494:refnum<visa-resource-name>)  [unwired: 7 in]
        n198 = call "DCIR_conf_alim.vi"("ErrIN"=w495, "VISAin"=w494) -> ("ErrOUT"=w492:errorcluster, "VisaOUT"=w486:refnum<visa-resource-name>)  [unwired: 8 in]
        n199 = Merge Errors(w492, w464) -> (w463:errorcluster)
        n200 = case shown="No Error" w463 {
          selector: w463 -> [w514 w551]
          tunnel: [w523 w552] -> w476
          tunnel: w486 -> [w522 _]
          tunnel: [w521 FALSE ("isPASS?")] -> w468
          tunnel: [w520 w552] -> w474
          tunnel: [w519 w551] -> w473
          tunnel: [w517 string[] [] ("tableau ajouté")] -> _
          tunnel: [w516 w550] -> _
          tunnel: [w515 w550] -> _
          tunnel: [w512 w550] -> w470
          tunnel: w469 -> [w511 _]
          tunnel: [w510 "" ("Chaîne")] -> w467
          tunnel: w461 -> [w497 _]
          tunnel: w460 -> [w496 _]
          frame No Error {
            n201 = call "DCIR_run_1pulseGene.vi"("3P4S"=w511, "Offset%"=sgl 0.0, "errin"=w514, "AmpCharg"=w496, "VisaAlimIn"=w522) -> ("errout"=w499:errorcluster, "DATAout"=w508:cluster{"Rch":dbl, "A ch":dbl, "max":dbl}, "VisaAlimOut"=w506:refnum<visa-resource-name>, "Out"=w518:T13, "Cell et DCIR ok"=w504:bool)  [unwired: 1 in, 1 out]
            n202 = local read "DCIR+?"() -> (w498:bool)
            n203 = call "Pico3-1pulse.vi"("+ ou -"=FALSE, "DataIn"=w508) -> ("Rout"=w516:string, "Chaîne"=w523:string)  [unwired: 8 in]
            n204 = call "Pico1-1.vi"("ajout test#"="Test# 6.5 - intradcir;", "Datain"=w518) -> ("taboutBdd"=w517:string[], "Chaîne"=w512:string)  [unwired: 8 in]
            n205 = Compound Arithmetic op=AND ("Opérateur arithmétique")(w498, invert w499) -> (w500:bool)
            n206 = case shown="True" w500 {
              tunnel: [w529 w547] -> w507
              tunnel: w506 -> [w530 w546]
              tunnel: [w530 w545] -> w505
              tunnel: [w527 w544] -> w503
              tunnel: w497 -> [_ w540]
              tunnel: w511 -> [_ w539]
              tunnel: [w524 w536] -> w510
              tunnel: w499 -> [w529 w535]
              tunnel: w498 -> [w528 _]
              tunnel: [w525 w533] -> w515
              tunnel: [w525 w532] -> w520
              frame False {
                w525 = "DCIR+ non executé" ("Chaîne")
                n207 = Not(x=w528) -> (.not. x?=w527:bool)
                n208 = Concatenate Strings(w525, "\r\n") -> (w524:string)
              }
              frame True {
                n209 = call "micro2.vi"("errin"=w535, "offset%"=25.0) -> ("errout"=w543:errorcluster)  [unwired: 9 in]
                n210 = call "DCIR_run_1pulseGene.vi"("3P4S"=w539, "Offset%"=sgl 50.0, "errin"=w543, "AmpCharg"=w540, "VisaAlimIn"=w546) -> ("errout"=w547:errorcluster, "DATAout"=w534:cluster{"Rch":dbl, "A ch":dbl, "max":dbl}, "VisaAlimOut"=w545:refnum<visa-resource-name>, "Out"=w538:T13, "Cell et DCIR ok"=w544:bool)  [unwired: 1 in, 1 out]
                n211 = call "Pico3-1pulse.vi"("+ ou -"=TRUE, "DataIn"=w534) -> ("Rout"=w533:string, "Chaîne"=w532:string)  [unwired: 8 in]
                n212 = call "Pico1-1.vi"("ajout test#"="Test# 6.6 - intradcir;", "Datain"=w538) -> ("Chaîne"=w536:string)  [unwired: 8 in, 1 out]
              }
            }
            n213 = local write "Chaîne"("Test DCIR: Puissance" ("Chaîne")) -> ()
            n214 = call <instrlib>:"Close.vi"("error in (no error)"=w507, "VISA resource name"=w505) -> ("error out"=w519:errorcluster)  [unwired: 9 in]
            n215 = And(x=w503, y=w504) -> (x .and. y?=w521:bool)
          }
          frame Error {
            w550 = "" ("Rout")
            w552 = "DCIR Skiped" ("Chaîne")
            n216 = One Button Dialog ("Boîte de dialogue à un bouton")(message="Initialisation de Hitech FAIL\nou lecture courant DCIR") -> ()  [unwired: 1 in, 1 out]
          }
        }
        n217 = local read "Config Path"() -> (w458:string)
        n218 = call "TestPostDCIR.vi"("Variante"=w458, "errin"=w473, "3P4S?"=w469, "isPASS?"=w468) -> ("errout"=w479:errorcluster, "message box"=w466:string, "test OK?"=→"Ok final":bool, "Chaîne 2"=w475:string, "offprbarre"=w471:bool)  [unwired: 2 in, 1 out]
        n219 = property on="progression" class="Slide (strict)"("Visible"=w471) -> ()  [unwired: 2 in, 2 out]
        n220 = local write "Chaîne"(w466) -> ()
        n221 = local read "UNO TAK out"() -> (w480:T2)
        n222 = Concatenate Strings(w476, w470, w474, w467, w475) -> (w489:string)
        n223 = call "Close TakTak.vi"("errin"=w479, "UNO Tak in"=w480) -> ("Error Out"=w462:errorcluster)  [unwired: 9 in]
        n224 = Write to Text File(file (use dialog)=w488, text=w489, error in=w491) -> (refnum out=w487:refnum<file>, error out=w490:errorcluster)  [unwired: 1 in, 1 out]
      }
      frame "Demontage" {
        # "On retire le Pack"
        n225 = Increment(x=w574) -> (x+1=w576:T8)
        n226 = call "Réponse Opérateur.vi"("errin"=w566, "expression régulière"="OUI|NON") -> ("errout"=w581:errorcluster, "toute l'expression"=w580:string)  [unwired: 7 in, 1 out]
        n227 = local write "image"("Deconnection stack") -> ()
        n228 = Equal?(x="OUI", y=w580) -> (x = y?=w578:bool)
        n229 = local read "Auto?"() -> (w560:bool)
        n230 = case shown="True" w578 {
          selector: w578 -> [w593 _]
          tunnel: w581 -> [w592 w594]
          tunnel: [w593 w597] -> w570
          tunnel: [w592 w600] -> w571
          frame False {
          }
          frame True {
            n231 = call "Réponse Opérateur.vi"("errin"=w594, "expression régulière"="OUI|NON") -> ("errout"=w600:errorcluster, "toute l'expression"=w598:string)  [unwired: 7 in, 1 out]
            n232 = local write "image"("Pack_remove") -> ()
            n233 = local write "Chaîne"("retirer le pack" ("chaîne")) -> ()
            n234 = Equal?(x="OUI", y=w598) -> (x = y?=w597:bool)
          }
        }
        n235 = local write "Chaîne"("retirer les connecteur de puissance" ("chaîne")) -> ()
        n236 = Select(t="Vérifiez bien que les voyants soient éteint" ("cas vrai"), s=w560, f="remettre le tiroir en position neutre" ("chaîne")) -> (s? t:f=w564:string)
        n237 = Select(t="TiroirCMDauto" ("cas vrai"), s=w560, f="TiroirCMD" ("chaîne")) -> (s? t:f=w559:string)
        n238 = case shown="True" w570 {
          selector: w570 -> [w584 _]
          tunnel: w571 -> [w583 _]
          tunnel: [w584 w587] -> w555
          tunnel: [w583 w590] -> w558
          tunnel: w564 -> [_ w586]
          tunnel: w559 -> [_ w585]
          frame False {
          }
          frame True {
            n239 = local write "Chaîne"(w586) -> ()
            n240 = local write "image"(w585) -> ()
            n241 = call "Réponse Opérateur.vi"("expression régulière"="OUI|NON") -> ("errout"=w590:errorcluster, "toute l'expression"=w588:string)  [unwired: 8 in, 1 out]
            n242 = Equal?(x="OUI", y=w588) -> (x = y?=w587:bool)
          }
        }
        n243 = local read "Ok final"() -> (w557:bool)
        n244 = And(x=w557, y=w555) -> (x .and. y?=w556:bool)
        n245 = Select(t=w576, s=w556, f=nav."CRASH") -> (s? t:f=w575:T8)
      }
      frame "CLOSE" {
        w627 = "Une autre pièce ?" ("chaîne")
        n246 = local read "Ok final"() -> (w616:bool)
        n247 = call "Réponse Opérateur.vi"("errin"=w626, "expression régulière"="OUI|NON") -> ("errout"=w611:errorcluster, "toute l'expression"=w633:string)  [unwired: 7 in, 1 out]
        n248 = local write "Chaîne"(w627) -> ()
        n249 = Select ("Sélectionner")(t="Next", s=w616, f="NextFAIL" ("cas faux")) -> (s? t:f=w624:string)
        n250 = local write "image"(w624) -> ()
        n251 = Concatenate Strings(w627, w633) -> (w634:string)
        n252 = Equal?(x=w633, y="OUI") -> (x = y?=w631:bool)
        n253 = call <userlib>:"Log_basic.vi"("errin"=w637, "chaîne"=w634, "in"=w636) -> ("sortie d'erreur"=w620:errorcluster, "refnum en sortie"=w621:refnum<file>)  [unwired: 7 in]
        n254 = local read "Config Path"() -> (w608:string)
        n255 = Close File(refnum=w621, error in=w620) -> (path=w613:path, error out=w619:errorcluster)
        n256 = Select(t=nav."DEM2", s=w631, f=nav."extinction") -> (s? t:f=w628:T8)
        n257 = call "micro path.vi"("Config"=w608) -> ("appended path"=w612:path)  [unwired: 10 in]
        n258 = call <userlib>:"waitXms.vi"("attente (ms)"=u32 500, "errin"=w619) -> ("errout"=w618:errorcluster)  [unwired: 13 in]
        n259 = Copy(8:w618, 10:w612, 11:w613) -> (0:w614:errorcluster)  [unwired: 2 in, 2 out]
        n260 = call "PV generator OP100.vi"("errin"=w614, "network"=w612, "path in"=w613) -> ("errout"=w603:errorcluster, "network out"=w610:path)  [unwired: 4 in, 3 out]
        "network out" <- w610
        n261 = call <userlib>:"waitXms.vi"("attente (ms)"=u32 700, "errin"=w603) -> ("errout"=w604:errorcluster)  [unwired: 13 in]
        n262 = call <userlib>:"POP_GOOGLE.vi"("error in"=w604, "chemin"=w610) -> ("error out"=w607:errorcluster)  [unwired: 8 in, 1 out]
        n263 = call <userlib>:"waitXms.vi"("attente (ms)"=u32 700, "errin"=w607) -> ("errout"=w606:errorcluster)  [unwired: 13 in]
        n264 = call "PrintMain.vi"("errin"=w606, "HTML PV path"=w610) -> ("errout"=w609:errorcluster)  [unwired: 9 in]
      }
      frame "extinction" {
        # "ICI ON éTeint TOUT  fin du programme ou il n'y a pas eu de probleme"
      }
      frame "CRASH", Default {
        # "Fin du programme ou il y a un probleme"
        n265 = local write "image"("Crash") -> ()
        n266 = Concatenate Strings("Fin du programme" ("chaîne")) -> (w667:string)
        n267 = call <userlib>:"Log_basic.vi"("errin"=w665, "chaîne"=w667, "in"=w664) -> ("sortie d'erreur"=w660:errorcluster, "refnum en sortie"=w659:refnum<file>)  [unwired: 7 in]
        n268 = Close File(refnum=w659, error in=w660) -> (path=w652:path, error out=w658:errorcluster)
        n269 = call <userlib>:"waitXms.vi"("attente (ms)"=u32 500, "errin"=w658) -> ("errout"=w657:errorcluster)  [unwired: 13 in]
        n270 = call "micro path.vi"() -> ("appended path"=w650:path)  [unwired: 11 in]
        n271 = local write "Chaîne"("Il semblerait que vous rencontriez un problem, veuillez prevenir le Team Leader" ("chaîne")) -> ()
        n272 = Copy(8:w657, 10:w650, 11:w652) -> (0:w653:errorcluster)  [unwired: 2 in, 2 out]
        n273 = call "PV generator OP100.vi"("errin"=w653, "network"=w650, "path in"=w652) -> ("errout"=w654:errorcluster, "network out"=w647:path)  [unwired: 4 in, 3 out]
        n274 = call <userlib>:"POP_GOOGLE.vi"("error in"=w654, "chemin"=w647) -> ("error out"=w646:errorcluster)  [unwired: 8 in, 1 out]
        n275 = flat-sequence {
          tunnel: [TRUE] -> w668
          tunnel: w646 -> [_]
          frame #0 {
          }
        }
        n276 = call <userlib>:"waitXms.vi"("attente (ms)"=u32 600, "errin"=w646) -> ("errout"=w645:errorcluster)  [unwired: 13 in]
        n277 = call "PrintMain.vi"("errin"=w645, "HTML PV path"=w647) -> ("errout"=w648:errorcluster)  [unwired: 9 in]
      }
      frame "Collage PAD" {
        n278 = call "Réponse Opérateur.vi"("errin"=w676, "expression régulière"="OUI|NON") -> ("errout"=w683:errorcluster, "toute l'expression"=w684:string)  [unwired: 7 in, 1 out]
        n279 = Equal?(x="OUI", y=w684) -> (x = y?=w685:bool)
        n280 = local write "Chaîne"("Basculer le plateau" ("chaîne")) -> ()
        n281 = local write "image"("Bascule_plateau") -> ()
        n282 = case shown="True" w685 {
          selector: w685 -> [w699 _]
          tunnel: w683 -> [w698 w702]
          tunnel: [w699 w703] -> w686
          tunnel: [w698 w706] -> w687
          frame False {
          }
          frame True {
            n283 = call "Réponse Opérateur.vi"("errin"=w702, "expression régulière"="OUI|NON") -> ("errout"=w706:errorcluster, "toute l'expression"=w704:string)  [unwired: 7 in, 1 out]
            n284 = local write "Chaîne"("Effectuer le nettoyage" ("chaîne")) -> ()
            n285 = local write "image"("Nettoyage") -> ()
            n286 = Equal?(x="OUI", y=w704) -> (x = y?=w703:bool)
          }
        }
        n287 = case shown="True" w686 {
          selector: w686 -> [w689 _]
          tunnel: w687 -> [w688 w692]
          tunnel: [w689 w693] -> w672
          tunnel: [w688 w696] -> w670
          frame False {
          }
          frame True {
            n288 = local write "Chaîne"("" ("chaîne")) -> ()
            n289 = call "Réponse Opérateur.vi"("errin"=w692, "expression régulière"="OUI|NON") -> ("errout"=w696:errorcluster, "toute l'expression"=w694:string)  [unwired: 7 in, 1 out]
            n290 = local write "image"("Opercule") -> ()
            n291 = Equal?(x="OUI", y=w694) -> (x = y?=w693:bool)
          }
        }
        n292 = Select(t=nav."Demontage", s=w672, f=nav."CRASH") -> (s? t:f=w677:T8)
      }
      frame "PreDCIR" {
        n293 = local read "Config Path"() -> (w708:string)
        n294 = local read "3P4S?"() -> (w711:bool)
        n295 = call "ComCMOD.vi"("Variante"=w708, "errin"=w721, "PostDCIR ?"=FALSE, "3P4S"=w711) -> ("errout"=w710:errorcluster, "test OK?"=w709:bool, "Out"=w724:T13)  [unwired: 5 in]
        n296 = call "Pico1-1.vi"("ajout test#"="Test# 1 - predcir;", "Datain"=w724) -> ("Chaîne"=w712:string)  [unwired: 8 in, 1 out]
        n297 = Write to Text File(file (use dialog)=w713, text=w712, error in=w716) -> (refnum out=w714:refnum<file>, error out=w715:errorcluster)  [unwired: 1 in, 1 out]
        n298 = Select(t=nav."OCVACIR", s=w709, f=nav."CRASH") -> (s? t:f=w718:T8)
      }
    }
    "fin" <- w20
    n299 = Wait (ms)(milliseconds to wait=u32 200 ("attente (ms)")) -> ()  [unwired: 1 out]
  }
  n300 = while {
    shift-right: ["image"] -> _
    shift-left: "CMODBOX" ("image") -> [w730]
    shift-left: "" ("image") -> [w731]
    stop <- w726 stop-if-true
    n301 = Not Equal?(x=w730, y=w731) -> (x != y?=w729:bool)
    n302 = global read "VG_progressBar.vi" "progression"() -> (→"progression":u8)
    n303 = Wait (ms)(milliseconds to wait=u32 50 ("attente (ms)")) -> ()  [unwired: 1 out]
    n304 = case shown="True" w729 {
      tunnel: "image" -> [_ w741]
      frame False {
      }
      frame True {
        n305 = call <vilib>:"Application Directory.vi"() -> ("Application Directory"=w737:path)
        n306 = Path To String(path=w737) -> (string=w738:string)
        n307 = Concatenate Strings(w738, "\\Image\\" ("chaîne"), w741, ".jpg" ("chaîne")) -> (w736:string)
        "chaîne concaténée" <- w736
        n308 = String To Path(string=w736) -> (path=w735:path)
        n309 = call <vilib>:"Read JPEG File.vi"("error in (no error)"=errorcluster {"status"=FALSE, "code"=0, "source"=""}, "path to JPEG file"=w735) -> ("error out"=→"errout":errorcluster, "image data"=w742:T14)  [unwired: 7 in, 1 out]
        n310 = call <vilib>:"Draw Flattened Pixmap.vi"("image data"=w742) -> ("new picture"=→"Image 2D":picture)  [unwired: 8 in]
      }
    }
    n311 = local read "fin"() -> (w726:bool)
  }
  n312 = Merge Errors(w13, w11) -> (→"errout":errorcluster)
